vi "Build Valid Account String.vi"(6 "Account Verified?":bool, 11 "Bank Account in":refnum<class "Bank Account.lvclass">) -> (3 "Bank Account out":refnum<class "Bank Account.lvclass">, 4 "Value":string)   [LabVIEW 2016, in "CLD Exam - ATM.lvlib" / "Bank Account.lvclass"]
uses:
  Bank Account.lvclass
  Bank Account.lvclass/Bank Account.ctl
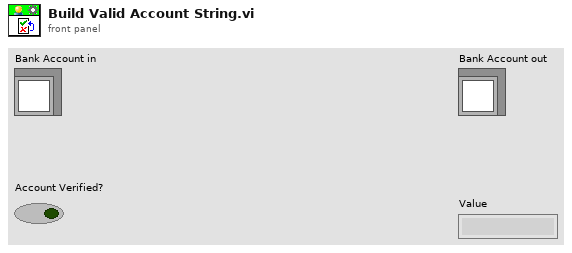
[diagram p1: front panel]
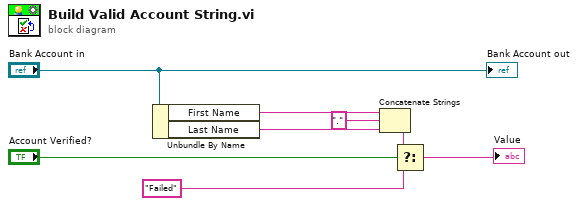
[diagram p0: block diagram]
diagram:
  n1 = Unbundle By Name("Bank Account in") -> ("First Name"=w6:string, "Last Name"=w5:string)
  n2 = Concatenate Strings(w6, "." ("string"), w5) -> (w2:string)
  n3 = Select(t=w2, s="Account Verified?", f="Failed") -> (s? t:f=→"Value":string)
  "Bank Account out" <- "Bank Account in"
